vi "Get Sensitivity.vi"(8 "error in (no error)":errorcluster, 11 "VISA resource name":refnum<visa-resource-name>) -> (0 "error out":errorcluster, 1 "Sensitivity (A or V)":dbl format="%#_6p", 2 "Sensitivty":string, 3 "VISA resource name out":refnum<visa-resource-name>)   [LabVIEW 2016, in "SR7270 Drivers.lvlib"]
uses:
  SR7270 Drivers.lvlib
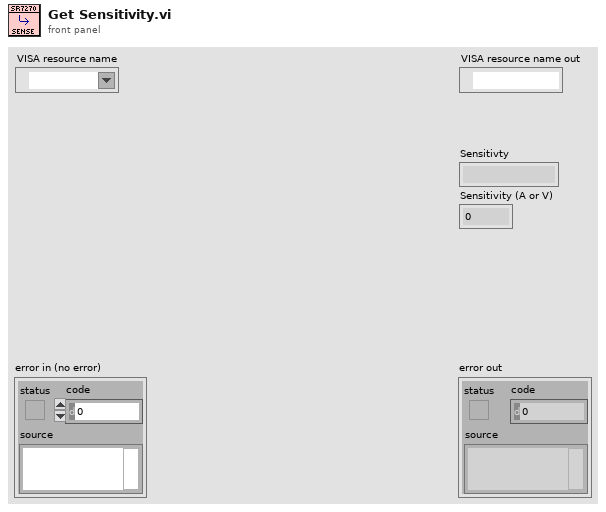
[diagram p1: front panel]
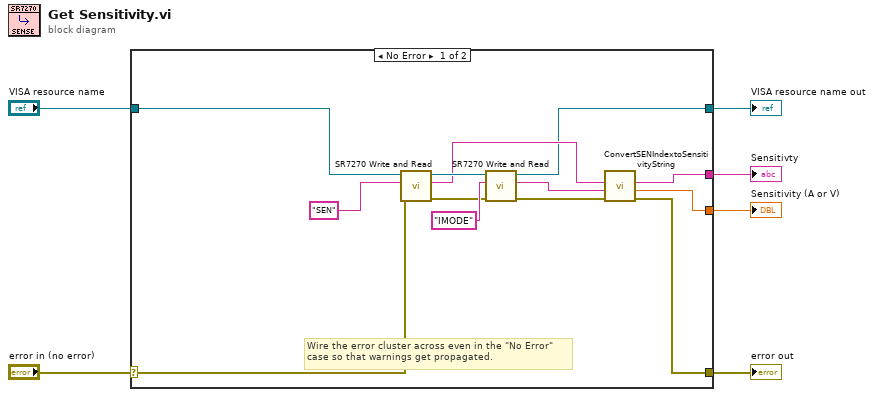
[diagram p0: block diagram]
diagram:
  n1 = case shown="No Error" "error in (no error)" {
    selector: "error in (no error)" -> [w19 w21]
    tunnel: [w11 w21] -> w5
    tunnel: [w7 w20] -> w3
    tunnel: "VISA resource name" -> [w8 w20]
    tunnel: [w10 _] -> w2
    tunnel: [w9 _] -> w1
    frame No Error {
      # "Wire the error cluster across even in the \"No Error\"\ncase so that warnings get propagated."
      n2 = call "SR7270 Write and Read.vi"("error in (no error)"=w19, "Command Name"="SEN", "VISA resource name"=w8) -> ("error out"=w12:errorcluster, "Read"=w15:string, "VISA resource name out"=w17:refnum<visa-resource-name>)  [unwired: 5 in, 1 out]
      n3 = call "SR7270 Write and Read.vi"("error in (no error)"=w12, "Command Name"="IMODE", "VISA resource name"=w17) -> ("error out"=w13:errorcluster, "Read"=w14:string, "VISA resource name out"=w7:refnum<visa-resource-name>)  [unwired: 5 in, 1 out]
      n4 = call "ConvertSENIndextoSensitivityString.vi"("error in (no error)"=w13, "IMODE"=w14, "SEN"=w15) -> ("error out"=w11:errorcluster, "Sensitivity (A or V)"=w9:dbl, "Sensitivty"=w10:string)  [unwired: 6 in]
    }
    frame Error {
    }
  }
  "error out" <- w5
  "VISA resource name out" <- w3
  "Sensitivty" <- w2
  "Sensitivity (A or V)" <- w1
